vi "DeInitialize.vi"(8 "error in (no error)":errorcluster, 11 "App in":refnum<class "App.lvclass">) -> (0 "error out":errorcluster, 3 "Shared.UI":refnum<class "UI.lvclass">)   [LabVIEW 2020, in "AR Example.lvlib" / "App.lvclass"]
uses:
  App.lvclass
  UI/UI.lvclass
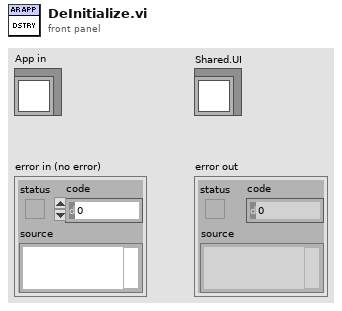
[diagram p1: front panel]
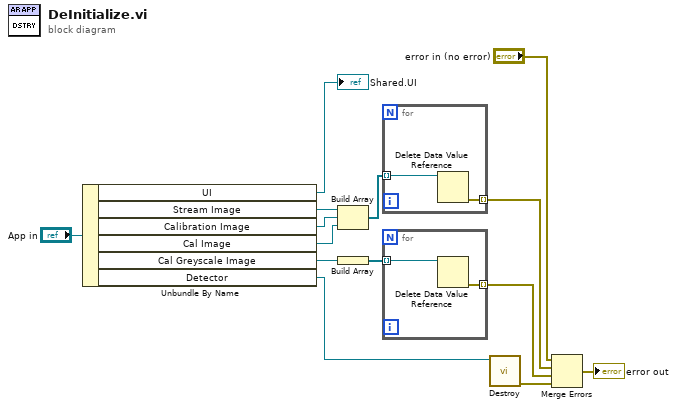
[diagram p0: block diagram]
diagram:
  n1 = Unbundle By Name("App in") -> ("UI"=→"Shared.UI":refnum<class "UI.lvclass">, "Stream Image"=w10:refnum<data-value>, "Calibration Image"=w9:refnum<data-value>, "Cal Image"=w4:refnum<data-value>, "Cal Greyscale Image"=w3:refnum<data-value>, "Detector"=w6:refnum<class "AprilTag Detector.lvclass">)
  n2 = Build Array(w10, w9, w4) -> (w8:refnum<data-value>[])
  n3 = Build Array(w3) -> (w2:refnum<data-value>[])
  n4 = for {
    tunnel: w8 -> [w16] mode=indexing
    tunnel: [w15] -> w7 mode=indexing
    n5 = Delete Data Value Reference(data value reference=w16) -> (error out=w15:errorcluster)  [unwired: 1 in, 1 out]
  }
  n6 = for {
    tunnel: w2 -> [w18] mode=indexing
    tunnel: [w17] -> w1 mode=indexing
    n7 = Delete Data Value Reference(data value reference=w18) -> (error out=w17:errorcluster)  [unwired: 1 in, 1 out]
  }
  n8 = call "Destroy.vi"("Apriltag Detector in"=w6) -> ("error out"=w5:errorcluster)  [unwired: 10 in]
  n9 = Merge Errors("error in (no error)", w7, w1, w5) -> (→"error out":errorcluster)
